vi "COB receive.vi"(6 "error in (no error)":errorcluster, 9 "CANopen in":refnum<class "CANopen.lvclass">) -> (0 "error out":errorcluster, 1 "No data?":bool, 2 "COB id":i32, 3 "CANopen out":refnum<class "CANopen.lvclass">, 4 "Data":u8[](array[numeric]))   [LabVIEW 2024, in "canopen.lvlib" / "CANopen.lvclass"]
doc: "Returns the oldest COB present in the reception queue."
uses:
  CANopen.lvclass
  CANopen.lvclass/CANopen.ctl
  HAL/HAL/Protocols/ICAN/ICAN.lvclass
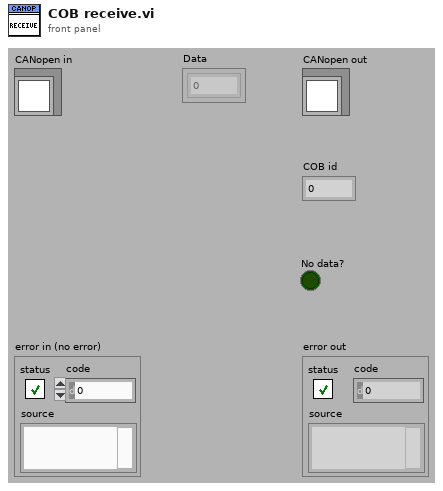
[diagram p1: front panel]
types:
  T1 = cluster{"ID":u32, "MSG type":u8, "DLC":u8, "Time Stamp":timestamp, "DATA":u8[]}
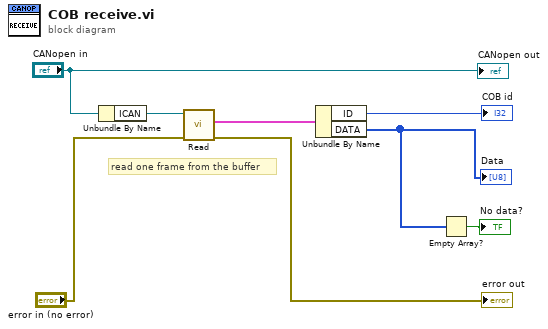
[diagram p0: block diagram]
diagram:
  # "read one frame from the buffer"
  n1 = Unbundle By Name("CANopen in") -> ("ICAN"=w8:refnum<class "ICAN.lvclass">)
  n2 = call-dynamic "Read.vi"("error in (no error)"="error in (no error)", "ICAN in"=w8) -> ("error out"=→"error out":errorcluster, "CAN Message"=w2:T1)  [unwired: 7 in, 1 out]
  n3 = Unbundle By Name(w2) -> ("ID"=→"COB id":u32, "DATA"=w1:u8[])
  "Data" <- w1
  n4 = Empty Array?(array=w1) -> (empty?=→"No data?":bool)
  "CANopen out" <- "CANopen in"
